vi "Dispose.vi"(8 "error in (no error)":errorcluster, 11 "FHPP in":refnum<class "FHPP.lvclass">) -> (0 "error out":errorcluster)   [LabVIEW 2022 SP3, in "FHPP.lvclass"]
uses:
  FHPP.lvclass
  FHPP.lvclass/FHPP.ctl
  <vilib>/Modbus/master/Modbus Master.lvclass
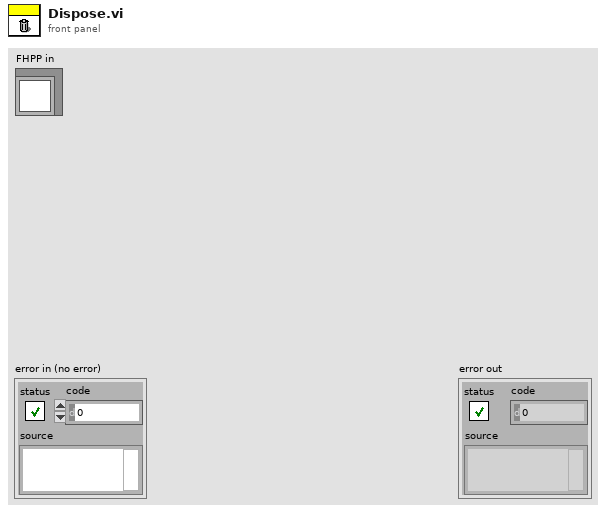
[diagram p1: front panel]
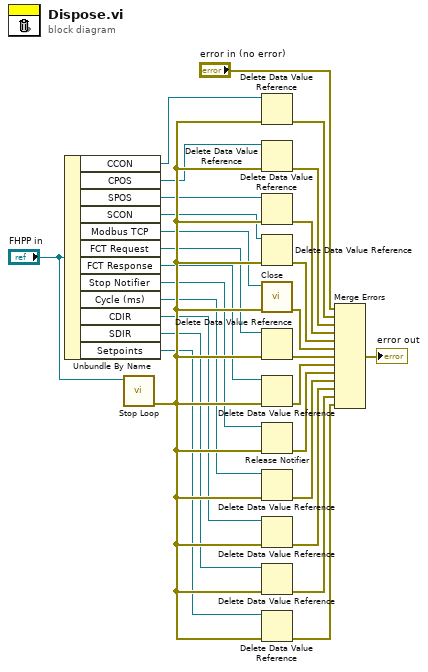
[diagram p0: block diagram]
diagram:
  n1 = Unbundle By Name("FHPP in") -> ("CCON"=w25:refnum<data-value>, "CPOS"=w24:refnum<data-value>, "SPOS"=w23:refnum<data-value>, "SCON"=w22:refnum<data-value>, "Modbus TCP"=w26:refnum<class "Modbus Master.lvclass">, "FCT Request"=w27:refnum<data-value>, "FCT Response"=w14:refnum<data-value>, "Stop Notifier"=w13:refnum<notifier>, "Cycle (ms)"=w9:refnum<data-value>, "CDIR"=w8:refnum<data-value>, "SDIR"=w7:refnum<data-value>, "Setpoints"=w3:refnum<data-value>)
  n2 = call "Stop Loop.vi"("FHPP in"="FHPP in") -> ("error out"=w28:errorcluster)  [unwired: 10 in]
  n3 = Delete Data Value Reference(data value reference=w25, error in=w28) -> (error out=w21:errorcluster)  [unwired: 1 out]
  n4 = Delete Data Value Reference(data value reference=w24, error in=w28) -> (error out=w20:errorcluster)  [unwired: 1 out]
  n5 = Delete Data Value Reference(data value reference=w23, error in=w28) -> (error out=w19:errorcluster)  [unwired: 1 out]
  n6 = Delete Data Value Reference(data value reference=w22, error in=w28) -> (error out=w18:errorcluster)  [unwired: 1 out]
  n7 = call-dynamic "Close.vi"("error in (no error)"=w28, "Modbus master in"=w26) -> ("error out"=w17:errorcluster)  [unwired: 9 in]
  n8 = Delete Data Value Reference(data value reference=w27, error in=w28) -> (error out=w12:errorcluster)  [unwired: 1 out]
  n9 = Delete Data Value Reference(data value reference=w14, error in=w28) -> (error out=w11:errorcluster)  [unwired: 1 out]
  n10 = Release Notifier(notifier=w13, error in (no error)=w28) -> (error out=w10:errorcluster)  [unwired: 1 in, 2 out]
  n11 = Delete Data Value Reference(data value reference=w9, error in=w28) -> (error out=w6:errorcluster)  [unwired: 1 out]
  n12 = Delete Data Value Reference(data value reference=w8, error in=w28) -> (error out=w5:errorcluster)  [unwired: 1 out]
  n13 = Delete Data Value Reference(data value reference=w7, error in=w28) -> (error out=w4:errorcluster)  [unwired: 1 out]
  n14 = Delete Data Value Reference(data value reference=w3, error in=w28) -> (error out=w2:errorcluster)  [unwired: 1 out]
  n15 = Merge Errors("error in (no error)", w21, w20, w19, w18, w17, w12, w11, w10, w6, w5, w4, w2) -> (→"error out":errorcluster)
